vi "Open Discovery Service Key File.vi"(8 "error in (no error)":errorcluster, 11 "Key File":path) -> (0 "error out":errorcluster, 3 "File Handle":i64)   [LabVIEW 2020, in "MeasurementLink Measurement Server.lvlib"]
uses:
  MeasurementLink Measurement Server.lvlib
  kernel32.dll
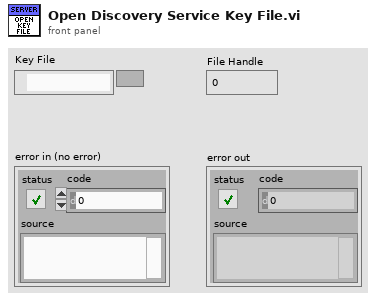
[diagram p1: front panel]
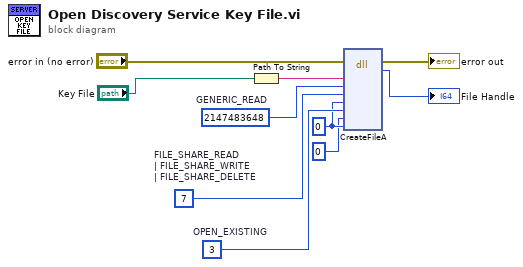
[diagram p0: block diagram]
diagram:
  w6 = i64 0 ("lpSecurityAttributes")
  w7 = u32 3  # OPEN_EXISTING
  w8 = u32 7  # FILE_SHARE_READ  | FILE_SHARE_WRITE  | FILE_SHARE_DELETE
  w9 = u32 2147483648  # GENERIC_READ
  n1 = Path To String(path="Key File") -> (string=w10:string)
  n2 = dll-call lib="kernel32.dll" fn="CreateFileA"(error in="error in (no error)", "lpFileName"=w10, "dwDesiredAccess"=w9, "dwShareMode"=w8, "lpSecurityAttributes"=w6, "dwCreationDisposition"=w7, "dwFlagsAndAttributes"=u32 0, "hTemplateFile"=w6) -> (error out=→"error out":errorcluster, "return type"=→"File Handle":i64)  [unwired: 9 in, 1 out]
